vi "Locate P2.vi"(0 "Image In":T2, 11 "Error In":errorcluster, 12 "Template File Path (P2 Hole)":path=path "C:/Users/serce/Desktop/Smart Vision System Testbench/P2 Hole Template.png") -> (1 "Number of Matches (P2 Hole)":i32, 3 "Coordinate System Out (Set Coordinate P2)":T1 {"Measurement System"."Axis Reference" items=["Direct", "Indirect"]; "Measurement System"."Angle (deg)" format="%.2f"; "Measurement System"."Origin"."Y" format="%.2f"; "Measurement System"."Origin"."X" format="%.2f"; "Reference System"."Axis Reference" items=["Direct", "Indirect"]; "Reference System"."Angle (deg)" format="%.2f"; "Reference System"."Origin"."Y" format="%.2f"; "Reference System"."Origin"."X" format="%.2f"}, 4 "Image Out":T2, 14 "Bounding Box":cluster{"x":sgl, "y":sgl}[](array[cluster]), 15 "Error Out":errorcluster)   [LabVIEW 2020]
uses:
  <vilib>/vision/Image Controls.llb/IMAQ Image.ctl
  <vilib>/vision/Pattern Matching.llb/IMAQ Curve Parameters.ctl
  <vilib>/vision/Pattern Matching.llb/IMAQ Match Range Setting.ctl
  <vilib>/vision/Pattern Matching.llb/IMAQ Geometric Pattern 2 Advanced Match Options.ctl
  <vilib>/vision/NI_Vision_Development_Module.lvlib
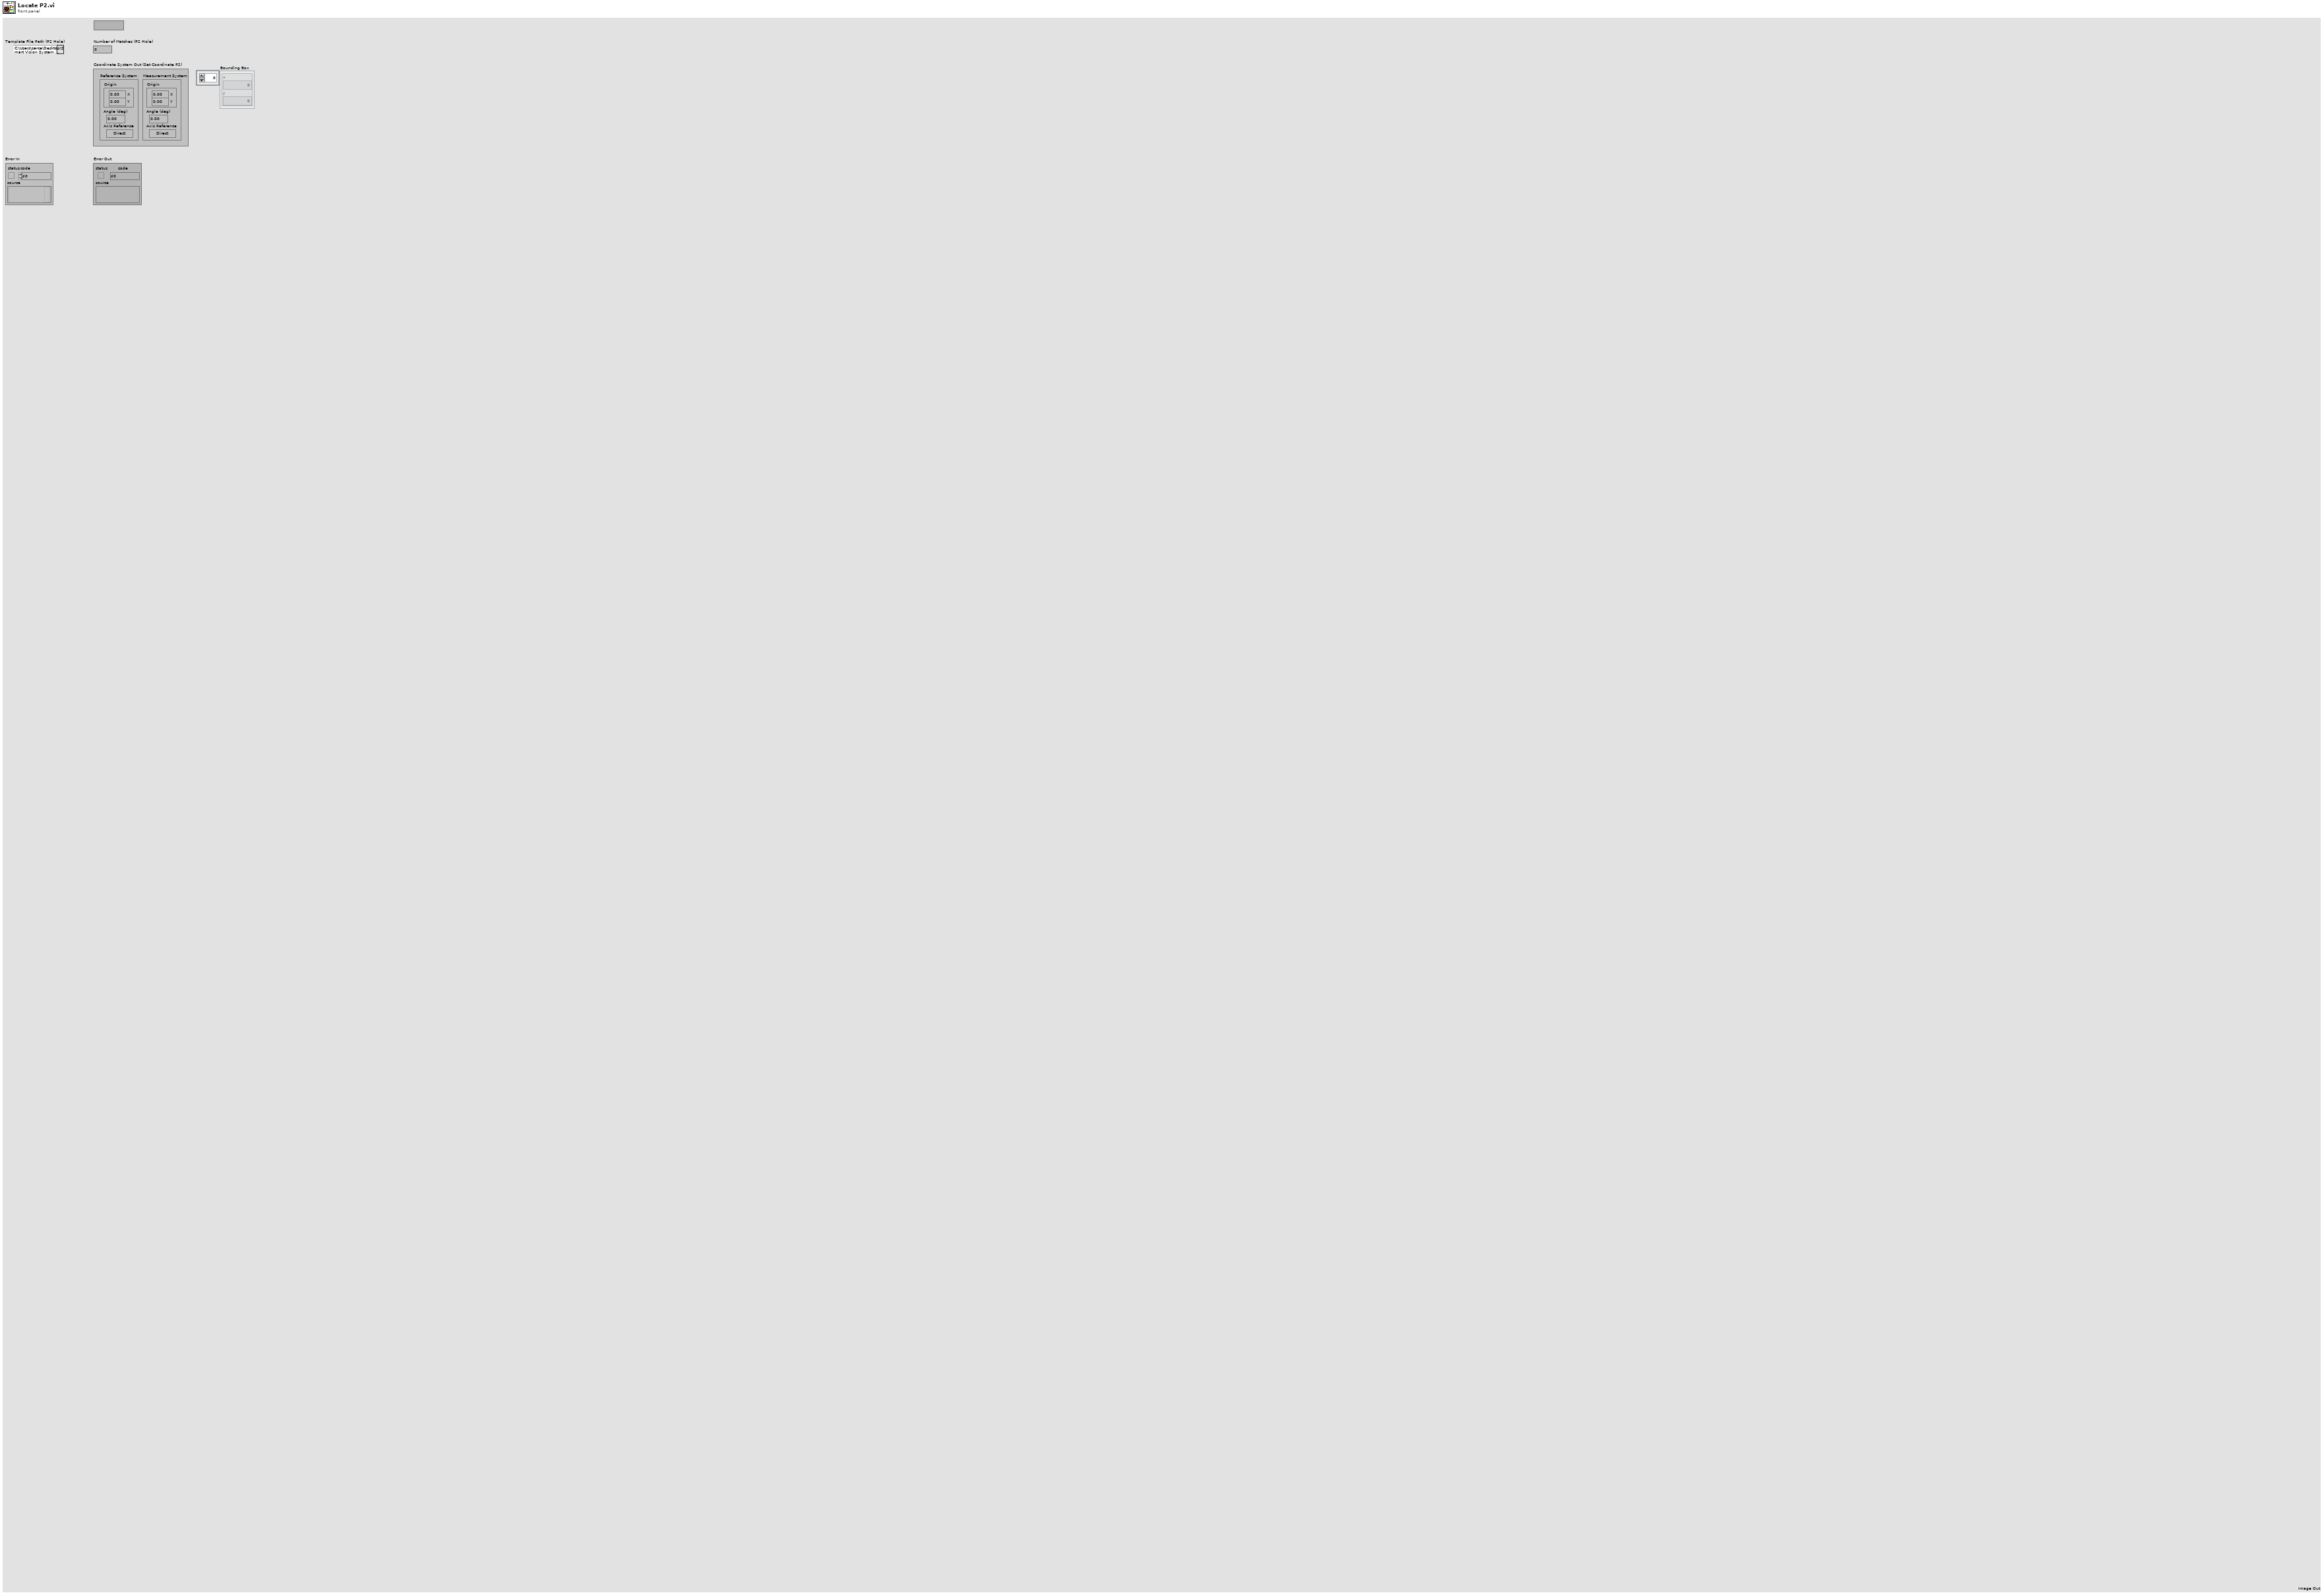
[diagram p1: front panel]
types:
  T1 = cluster{"Reference System":cluster{"Origin":cluster{"X":sgl, "Y":sgl}, "Angle (deg)":sgl, "Axis Reference":u32}, "Measurement System":cluster{"Origin":cluster{"X":sgl, "Y":sgl}, "Angle (deg)":sgl, "Axis Reference":u32}}
  T2 = typedef "IMAQ Image.ctl" = refnum<image>
  T3 = enum16{"Reset", "Update Coordinate System", "Get Coordinate System"}
  T4 = enum16{"Horizontal Motion", "Vertical Motion", "Horizontal and Vertical Motion", "Horizontal, Vertical and Angular Motion"}
  T5 = cluster{"Origin":cluster{"X":sgl, "Y":sgl}, "Angle (deg)":sgl, "Axis Reference":u32}
  T6 = typedef "IMAQ Curve Parameters.ctl" = cluster{"Extraction Mode":u32, "Edge Threshold":i32, "Edge Filter Size":u32, "Min Length":i32, "Row Search Step Size":i32, "Col Search Step Size":i32, "Max Endpoint Gap":i32, "Closed":bool, "Subpixel":bool}
  T7 = typedef "IMAQ Match Range Setting.ctl" = cluster{"Match Constraints":u32, "Min":dbl, "Max":dbl}
  T8 = typedef "IMAQ Geometric Pattern 2 Advanced Match Options.ctl" = u16
  T9 = cluster{"Curve Parameters":T6, "Match Mode":cluster{"Rotation":bool, "Scale":bool, "Occlusion":bool, "Reserved 1":bool, "Reserved 2":bool, "Reserved 3":bool}, "Range Settings":T7[], "Number of Matches":i32, "Minimum Match Score":sgl, "SubPixel Accuracy":bool, "Adv. Geometric Match Options 2":cluster{"Setup Data Item":T8, "Item Value":dbl}[]}
  T10 = cluster{"Global Rectangle":i32[], "Contours":cluster{"ID":enum32{"External", "Internal"}, "Type":u32, "Coordinates":i32[]}[]}
  T11 = cluster{"Brightness":sgl, "Contrast":sgl, "Gamma":sgl}
  T12 = typedef "IMAQ GM Match Report.ctl" = cluster{"Position":cluster{"x":sgl, "y":sgl}, "Angle":sgl, "Scale":sgl, "Score":sgl, "Bounding Box":cluster{"x":sgl, "y":sgl}[], "Contrast Reversed":bool, "Occlusion %":sgl, "Template Target Curve Score":sgl, "Target Template Curve Score":sgl, "Correlation Score":sgl}
  T13 = typedef "IMAQ Coordinate System" = cluster{"Reference System":cluster{"Origin":cluster{"X":sgl, "Y":sgl}, "Angle (deg)":sgl, "Axis Reference":u32}, "Measurement System":cluster{"Origin":cluster{"X":sgl, "Y":sgl}, "Angle (deg)":sgl, "Axis Reference":u32}}
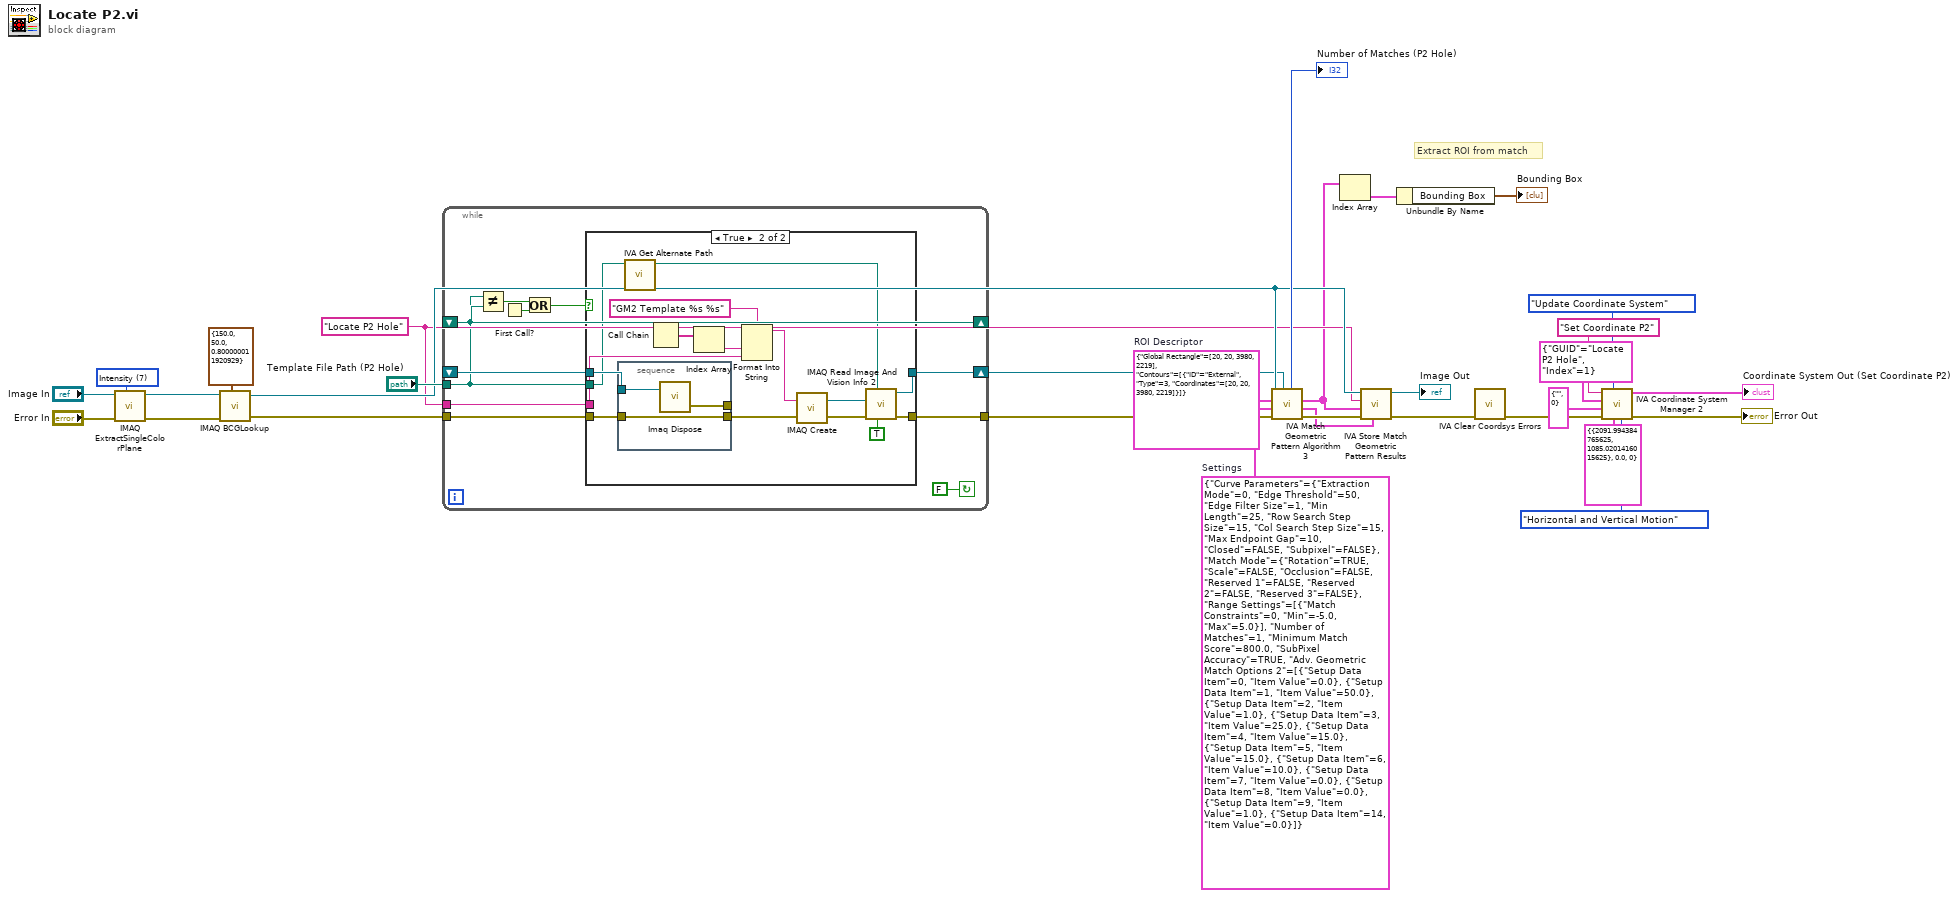
[diagram p0: block diagram]
diagram:
  w5 = 7 items=["Red", "Green", "Blue", "Hue", "Saturation", "Luminance", "Value", "Intensity"] ("Color Plane")
  w23 = T9 {"Curve Parameters"={"Extraction Mode"=0, "Edge Threshold"=50, "Edge Filter Size"=1, "Min Length"=25, "Row Search Step Size"=15, "Col Search Step Size"=15, "Max Endpoint Gap"=10, "Closed"=FALSE, "Subpixel"=FALSE}, "Match Mode"={"Rotation"=TRUE, "Scale"=FALSE, "Occlusion"=FALSE, "Reserved 1"=FALSE, "Reserved 2"=FALSE, "Reserved 3"=FALSE}, "Range Settings"=[{"Match Constraints"=0, "Min"=-5.0, "Max"=5.0}], "Number of Matches"=1, "Minimum Match Score"=800.0, "SubPixel Accuracy"=TRUE, "Adv. Geometric Match Options 2"=[{"Setup Data Item"=0, "Item Value"=0.0}, {"Setup Data Item"=1, "Item Value"=50.0}, {"Setup Data Item"=2, "Item Value"=1.0}, {"Setup Data Item"=3, "Item Value"=25.0}, {"Setup Data Item"=4, "Item Value"=15.0}, {"Setup Data Item"=5, "Item Value"=15.0}, {"Setup Data Item"=6, "Item Value"=10.0}, {"Setup Data Item"=7, "Item Value"=0.0}, {"Setup Data Item"=8, "Item Value"=0.0}, {"Setup Data Item"=9, "Item Value"=1.0}, {"Setup Data Item"=14, "Item Value"=0.0}]}  # Settings
  w22 = "Locate P2 Hole" ("Step Name")
  w29 = T10 {"Global Rectangle"=[20, 20, 3980, 2219], "Contours"=[{"ID"=enum."External", "Type"=3, "Coordinates"=[20, 20, 3980, 2219]}]}  # ROI Descriptor
  # "Extract ROI from match"
  n1 = call "IMAQ ExtractSingleColorPlane"("Color Plane"=w5, "error in (no error)"="Error In", "Image Src"="Image In") -> ("error out"=w1:errorcluster, "Image Dst Out"=w2:T2)  [unwired: 7 in]
  n2 = call "IMAQ BCGLookup"("Image Src"=w2, "BCG Values"=T11 {"Brightness"=150.0, "Contrast"=50.0, "Gamma"=0.8}, "error in (no error)"=w1) -> ("Image Dst Out"=w24:T2, "error out"=w25:errorcluster)  [unwired: 2 in, 2 out]
  n3 = while {
    shift-right: [w42] -> w20
    shift-left: _ -> [w41]
    tunnel: [w39] -> w21
    tunnel: w25 -> [w38]
    tunnel: "Template File Path (P2 Hole)" -> [w32]
    tunnel: w22 -> [w37]
    shift-right: [w32] -> _
    shift-left: _ -> [w36]
    stop <- FALSE continue-if-true
    n4 = Not Equal?(x=w32, y=w36) -> (x != y?=w34:bool)
    n5 = First Call?() -> (First Call?: T/F=w35:bool)
    n6 = Or(x=w34, y=w35) -> (x .or. y?=w33:bool)
    n7 = case shown="True" w33 {
      tunnel: [w44 w46] -> w42
      tunnel: w41 -> [w44 w53]
      tunnel: [w43 w48] -> w39
      tunnel: w38 -> [w43 w54]
      tunnel: w37 -> [_ w55]
      tunnel: w32 -> [_ w52]
      frame False {
      }
      frame True {
        n8 = stacked-sequence {
          tunnel: w54 -> [w62]
          tunnel: w53 -> [w61]
          tunnel: [w62] -> w51
          tunnel: [w60] -> _
          frame #0 {
            n9 = call "Imaq Dispose"("Image"=w61) -> ("error out"=w60:errorcluster)  [unwired: 2 in, 3 out]
          }
        }
        n10 = call <vilib>:"IVA Get Alternate Path.vi"("Path In"=w52) -> ("Path Out"=w47:path)  [unwired: 10 out]
        n11 = Call Chain() -> (call chain=w57:string[])
        n12 = Index Array(array=w57) -> (element=w56:string)  [unwired: 1 in]
        n13 = Format Into String(format string="GM2 Template %s %s" ("Image Name"), w56, w55) -> (resulting string=w59:string)  [unwired: 2 in, 1 out]
        n14 = call "IMAQ Create"("Image Name"=w59, "error in (no error)"=w51) -> ("New Image"=w45:T2, "error out"=w49:errorcluster)  [unwired: 2 in, 1 out]
        n15 = call "IMAQ Read Image And Vision Info 2"("Use File Path Image Type"=TRUE, "File Path"=w47, "error in (no error)"=w49, "Image"=w45) -> ("error out"=w48:errorcluster, "Image Out"=w46:T2)  [unwired: 5 in, 1 out]
      }
    }
  }
  n16 = call <vilib>:"IVA Match Geometric Pattern Algorithm 3.vi"("Template"=w20, "error in (no error)"=w21, "Settings"=w23, "ROI Descriptor"=w29, "Image"=w24) -> ("error out"=w28:errorcluster, "Calibrated Matches"=w27:T12[], "Matches"=w8:T12[], "Number of Matches"=→"Number of Matches (P2 Hole)":i32)  [unwired: 3 out]
  n17 = Index Array(array=w8) -> (element=w7:T12)  [unwired: 1 in]
  n18 = call <vilib>:"IVA Store Match Geometric Pattern Results.vi"("Calibrated Matches"=w27, "error in (no error)"=w28, "Matches"=w8, "Step Name"=w22, "Image in"=w24) -> ("error out"=w19:errorcluster, "Image dup"=→"Image Out":T2)  [unwired: 5 out]
  n19 = Unbundle By Name(w7) -> ("Bounding Box"=→"Bounding Box":cluster{"x":sgl, "y":sgl}[])
  n20 = call <vilib>:"IVA Clear Coordsys Errors.vi"("error in (no error)"=w19) -> ("error out"=w11:errorcluster)  [unwired: 10 in]
  n21 = call <vilib>:"IVA Coordinate System Manager 2.vi"("Mode"=T4."Horizontal and Vertical Motion", "Reference System"=T5 {"Origin"={"X"=2091.9944, "Y"=1085.0201}, "Angle (deg)"=0.0, "Axis Reference"=0}, "Function"=T3."Update Coordinate System", "error in (no error)"=w11, "Angle ID"=cluster{"GUID":string, "Index":i32} {"GUID"="", "Index"=0}, "Origin ID"=cluster{"GUID":string, "Index":i32} {"GUID"="Locate P2 Hole", "Index"=1}, "Coordinate System Name"="Set Coordinate P2") -> ("error out"=→"Error Out":errorcluster, "Coordinate System Out"=→"Coordinate System Out (Set Coordinate P2)":T13)  [unwired: 3 out]
